vi "Get Title.vi"(8 "error in (no error)":errorcluster, 11 "AB_UI_Fmwrk_Build in":refnum<class "AB_UI_Frmwk_Build.lvclass">) -> (0 "error out":errorcluster, 2 "title":string, 3 "AB_UI_Fmwrk_Build out":refnum<class "AB_UI_Frmwk_Build.lvclass">)   [LabVIEW 2020, in "AB_UI_Frmwk_Build.lvclass"]
uses:
  <vilib>/AppBuilder/AB_Classes/Build/UI/AB_UI_Frmwk_Build.lvclass
  <vilib>/AppBuilder/AB_Classes/Build/AB_Build.lvclass
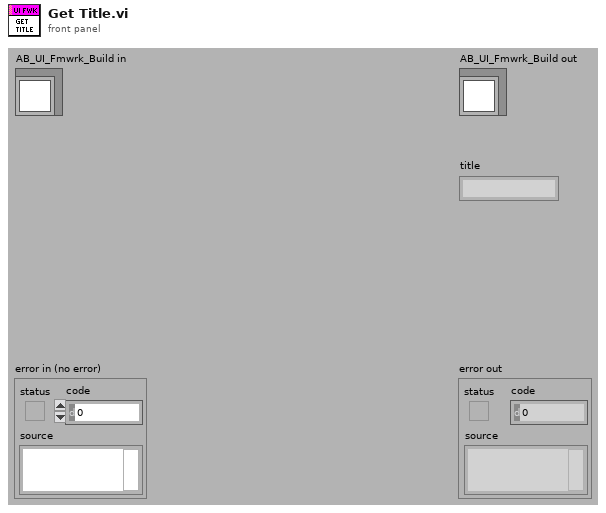
[diagram p1: front panel]
types:
  T1 = typedef "AB_Build.ctl" = cluster{"buildSpecName":string, "buildSpecDescription":string, "destinations":refnum<class "AB_Destination.lvclass">[], "exclusionOption":T2, "defaultLanguage":string, "supportedLanguages":string[], "excludedDirectories":path[], "buildContext":refnum<vi>, "buildObject":T3, "preview":bool, "programatic":bool, "progressBarEvents":T4, "userLog_Path":path, "preActionID":string, "preAction_Path":path, "postActionID":string, "postAction_Path":path, "eng_checkForBrokenVIs?":bool, "eng_verboseLinkerErrors?":bool, "localDest_Path":path, "targetDest_Path":path, "removeVIObject":u16, "cache":refnum<class "PreviewCache.lvclass">, "use cache":bool, "previewCache_ID":string, "buildCache_ID":string, "eng_TempLocalDest_Path":path, "eng_collectDependencies?":bool, "versionInfo":cluster{"buildVersion":cluster{"major":u16, "minor":u16, "patch":u16, "build":u16}, "autoIncrement":bool}, "eng_enableVIChecksums":bool}
  T2 = typedef "AB_Exclusion_Option.ctl" = cluster{"typedefs":bool, "polymorphicVIs":bool, "unusedLibraryItems":bool, "modifyLibraryFile":bool, "edit-timeDependencies":bool, "inlineVIs":bool, "dependent PPLs":bool, "dependent DLLs":bool}
  T3 = typedef "ItemRef.ctl" = u64
  T4 = typedef "provcom_ProgressBar_Events.ctl" = cluster{"newJob":refnum<user-event>, "newItem":refnum<user-event>, "errorMsg":T5, "cancel":refnum<user-event>}
  T5 = typedef "mxLvBuildError.ctl" = refnum<user-event>
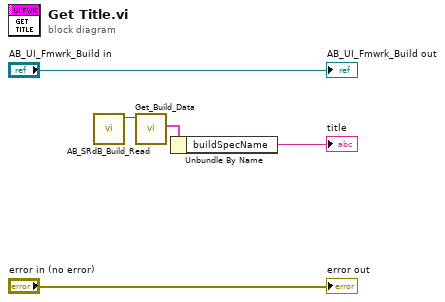
[diagram p0: block diagram]
diagram:
  n1 = call <resource>:"AB_SRdB_Build_Read.vi"() -> ("build out"=w4:refnum<class "AB_Build.lvclass">)  [unwired: 1 in, 10 out]
  n2 = call <vilib>:"Get_Build_Data.vi"("Class in"=w4) -> ("data"=w5:T1)  [unwired: 1 in, 9 out]
  n3 = Unbundle By Name(w5) -> ("buildSpecName"=→"title":string)
  "error out" <- "error in (no error)"
  "AB_UI_Fmwrk_Build out" <- "AB_UI_Fmwrk_Build in"
